vi "RePrint_Barcode.vi"(8 "error in":errorcluster, 9 "User Data":T1, 10 "RFID":string, 11 "Ref in":T2={"MS SQL Connection"=refnum, "UDL File"=path "", "Time"="", "DCODE"="", "WIP+1"=0, "MC No?"=0, "POKAYOKE?"=FALSE, "Expected Result"="", "Result [Status]"="", "Clock"=0.0, "RFID"="", "WIP Queue"=refnum, "TS Parameter"={"ProfitCenterCode"="", "LineCode"="", "WorkOrderNumber"="", "Model"="", "Model_with_Prefix"="", "VendorCode"="", "SetParameterDateCode"="", "PokaYoke"=0, "Target"=1, "Live_DateCode"="", "CustomerPartNumber"="", "Hand"="", "sBarcode"=FALSE, "FCA"=0, "Ent_Stamp"=timestamp(0 s since 1904-01-01), "STS_CD"=0.0}, "Data_Queue"=[], "RFID Serial No."=""} {"TS Parameter"."FCA" format="%01d"; "TS Parameter"."Target" min=1 max=100000; "TS Parameter"."PokaYoke" min=0 max=1}) -> (0 "error out":errorcluster, 2 "Barcode":string)   [LabVIEW 2020]
uses:
  Controls/TS_Parameter_V2.ctl
  Controls/TD SQL.ctl
  <vilib>/addons/database/Connection.llb/Conn ObjectReference.ctl
  Controls/WIP_State.ctl
  Controls/TS_Parameter.ctl
  Controls/user_log.ctl
  <vilib>/addons/database/Connection.llb/Conn Execute.vi
  MS SQL/MS_Global.vi
  <vilib>/addons/database/NI_Database_API.lvlib
panel:
  out "Total Seconds":i32
  out "TS Parameter":T5={"ProfitCenterCode"="", "LineCode"="", "WorkOrderNumber"="", "Model"="", "Model_with_Prefix"="", "VendorCode"="", "SetParameterDateCode"="", "PokaYoke"=0, "Target"=1, "Live_DateCode"="", "CustomerPartNumber"="", "Hose_Type"="", "sBarcode"=FALSE, "FCA"=0, "Ent_Stamp"=timestamp(0 s since 1904-01-01), "STS_CD"=0.0} {"FCA" format="%01d"; "Target" min=1 max=100000; "PokaYoke" min=0 max=1}
  out "text":string
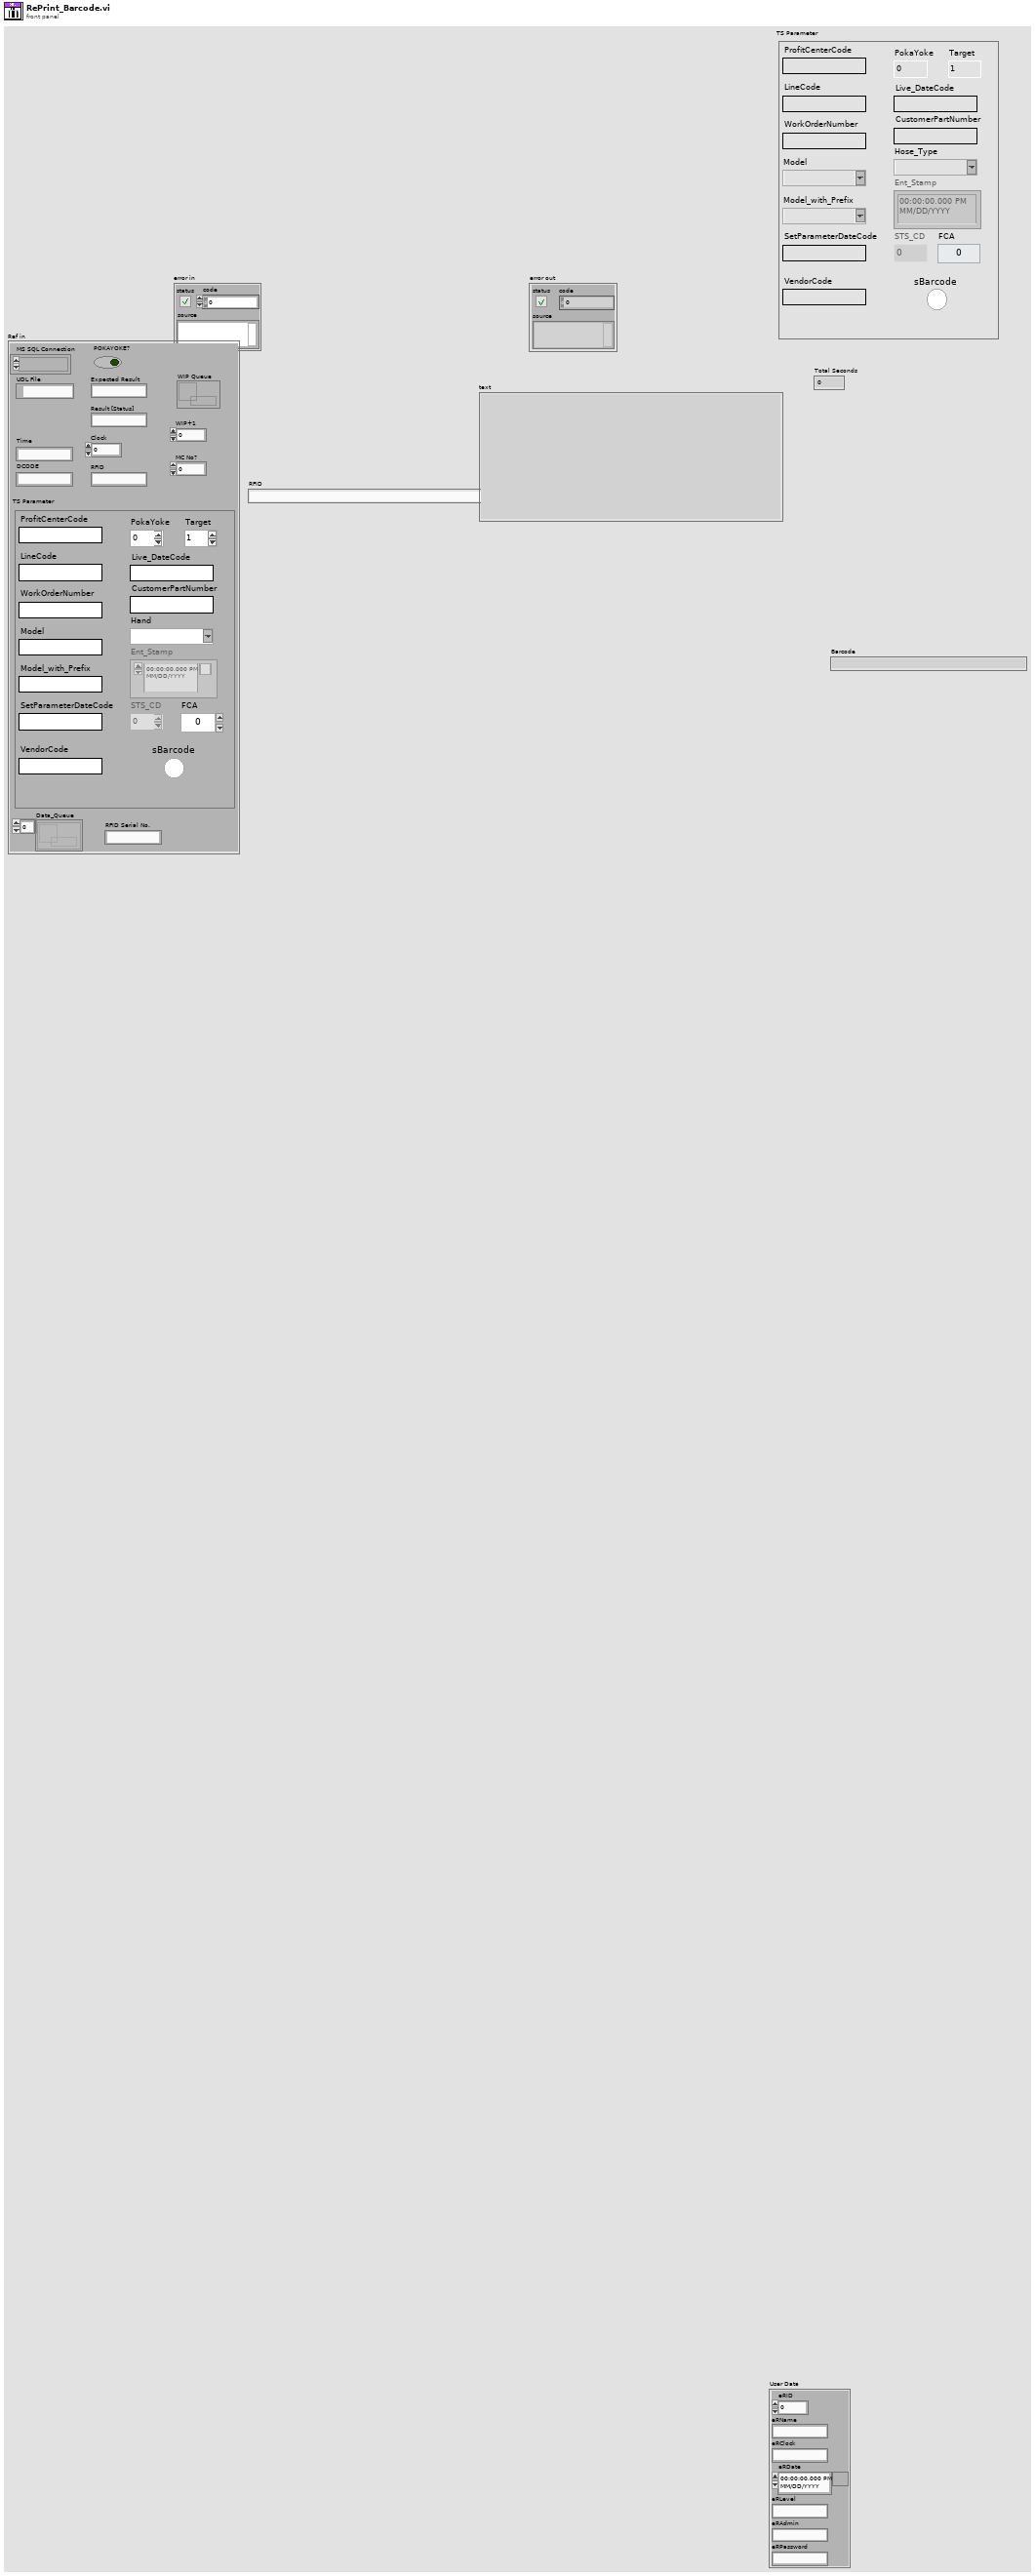
[diagram p1: front panel]
types:
  T1 = typedef "user_log.ctl" = cluster{"eRID":u16, "eRName":string, "eRClock":string, "eRDate":timestamp, "eRLevel":string, "eRAdmin":string, "eRPassword":string}
  T2 = typedef "TD SQL.ctl" = cluster{"MS SQL Connection":T3, "UDL File":path, "Time":string, "DCODE":string, "WIP+1":i64, "MC No?":i32, "POKAYOKE?":bool, "Expected Result":string, "Result [Status]":string, "Clock":dbl, "RFID":string, "WIP Queue":refnum<queue>, "TS Parameter":T4, "Data_Queue":refnum<queue>[], "RFID Serial No.":string}
  T3 = typedef "NI_Database_API.lvlib/Conn ObjectReference.ctl" = refnum<k1>
  T4 = typedef "TS_Parameter.ctl" = cluster{"ProfitCenterCode":string, "LineCode":string, "WorkOrderNumber":string, "Model":string, "Model_with_Prefix":string, "VendorCode":string, "SetParameterDateCode":string, "PokaYoke":i32, "Target":i32, "Live_DateCode":string, "CustomerPartNumber":string, "Hand":string, "sBarcode":bool, "FCA":i32, "Ent_Stamp":timestamp, "STS_CD":dbl}
  T5 = typedef "TS_Parameter_V2.ctl" = cluster{"ProfitCenterCode":string, "LineCode":string, "WorkOrderNumber":string, "Model":string, "Model_with_Prefix":string, "VendorCode":string, "SetParameterDateCode":string, "PokaYoke":i32, "Target":i32, "Live_DateCode":string, "CustomerPartNumber":string, "Hose_Type":string, "sBarcode":bool, "FCA":i32, "Ent_Stamp":timestamp, "STS_CD":dbl}
  T6 = enum16{"open", "replace", "create", "open or create", "replace or create", "replace or create with confirmation"}
  T7 = typedef "LVDateTimeRec.ctl" = cluster{"fractional second":dbl, "second":i32, "minute":i32, "hour":i32, "day of month":i32, "month":i32, "year":i32, "day of week":i32, "day of year":i32, "DST":i32}
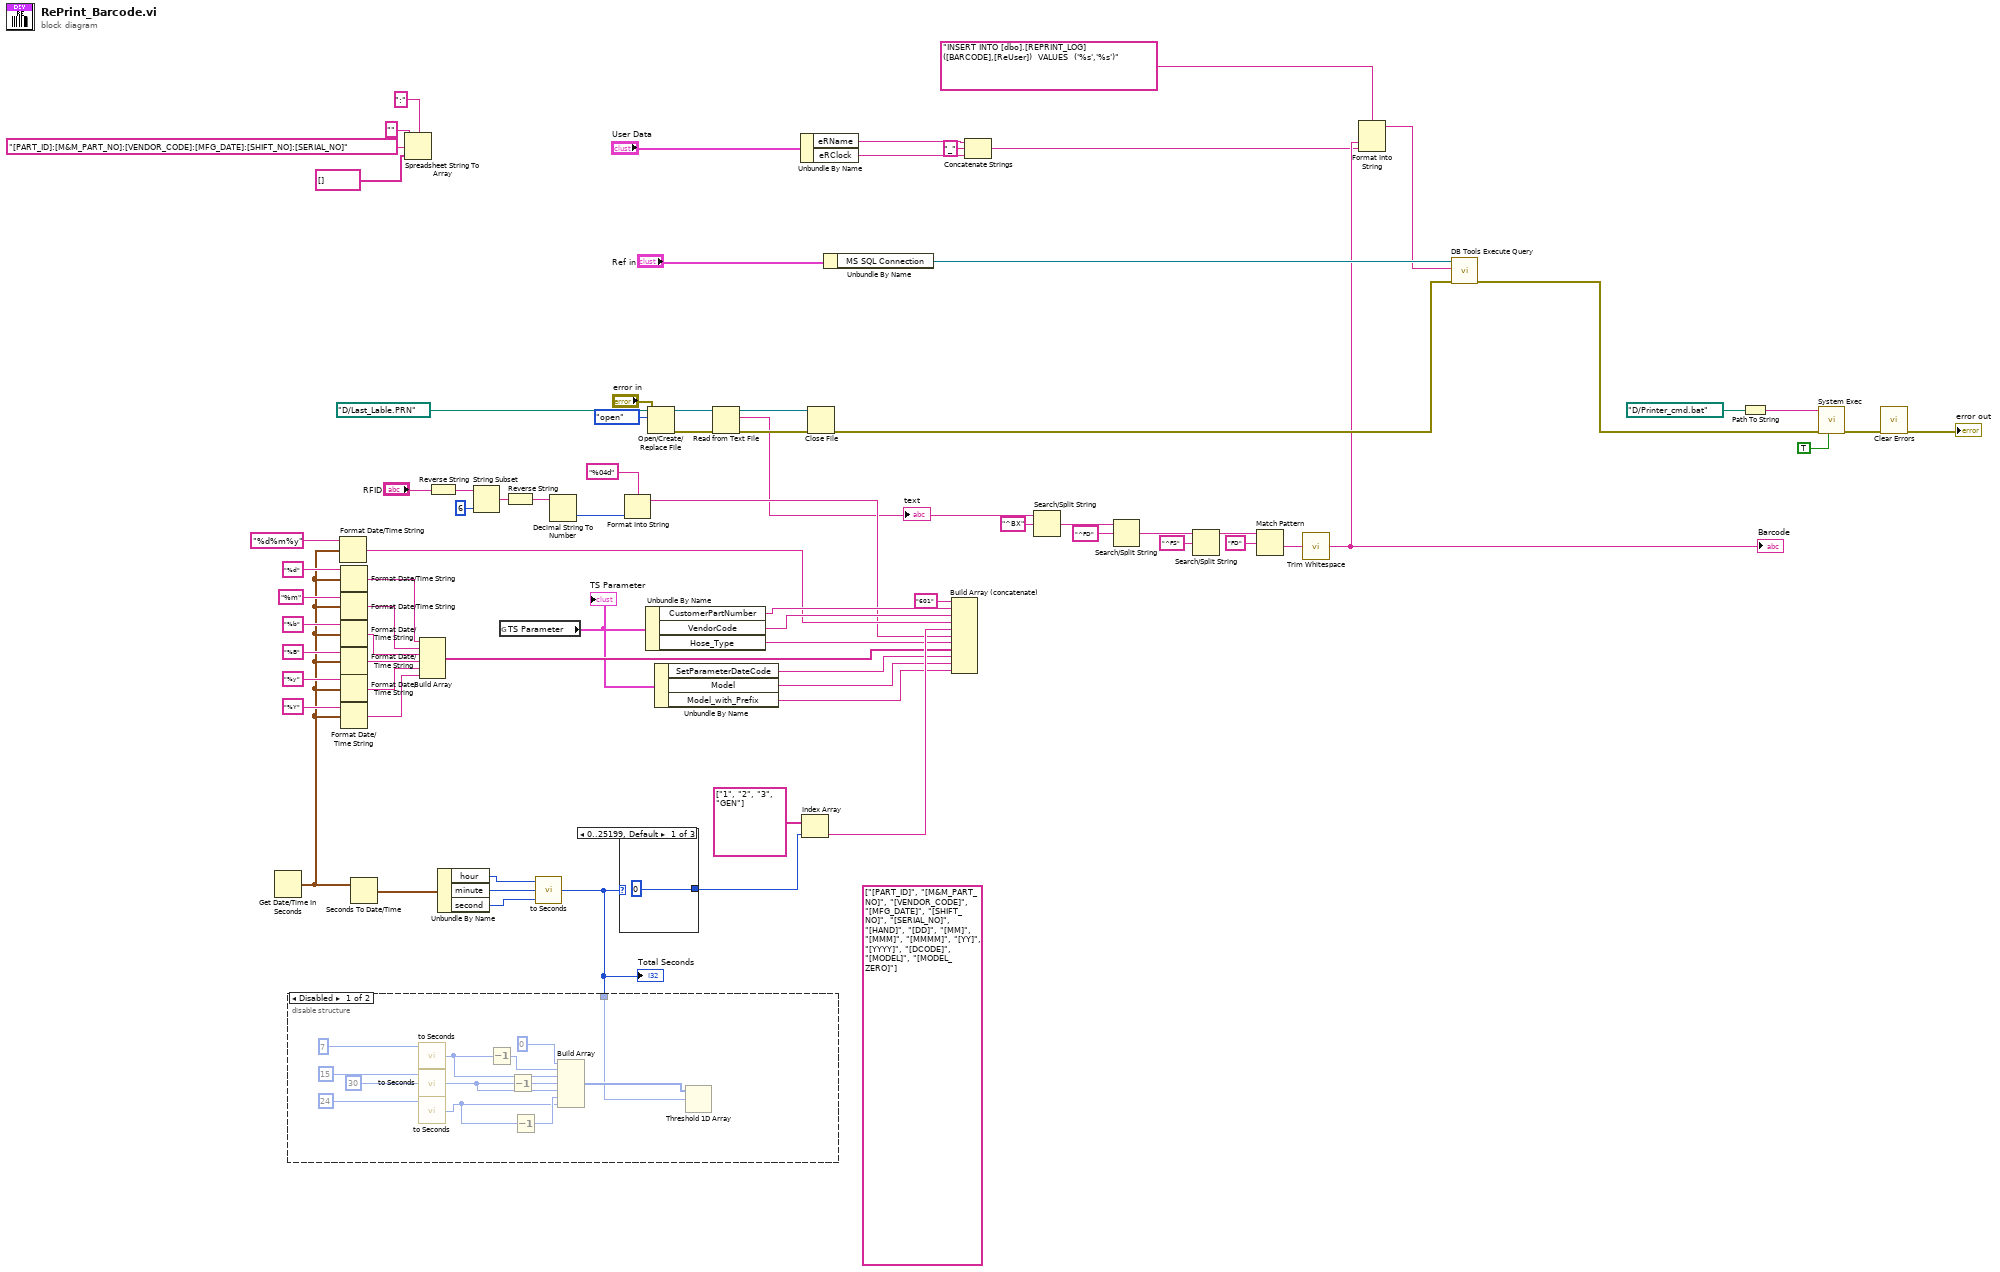
[diagram p0: block diagram]
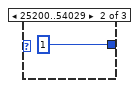
[diagram p3: hidden frame]
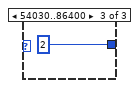
[diagram p4: hidden frame]
diagram:
  (unwired) string[] ["[PART_ID]", "[M&M_PART_NO]", "[VENDOR_CODE]", "[MFG_DATE]", "[SHIFT_NO]", "[SERIAL_NO]", "[HAND]", "[DD]", "[MM]", "[MMM]", "[MMMM]", "[YY]", "[YYYY]", "[DCODE]", "[MODEL]", "[MODEL_ZERO]"] ("array")
  n1 = Get Date/Time In Seconds() -> (seconds since 1Jan1904=w33:timestamp)
  n2 = Format Date/Time String(time format string (%c)="%d%m%y", seconds (now)=w33) -> (date/time string=w64:string)  [unwired: 1 in]
  n3 = Format Date/Time String(time format string (%c)="%d", seconds (now)=w33) -> (date/time string=w46:string)  [unwired: 1 in]
  n4 = Format Date/Time String(time format string (%c)="%m", seconds (now)=w33) -> (date/time string=w45:string)  [unwired: 1 in]
  n5 = Format Date/Time String(time format string (%c)="%b", seconds (now)=w33) -> (date/time string=w44:string)  [unwired: 1 in]
  n6 = Format Date/Time String(time format string (%c)="%B", seconds (now)=w33) -> (date/time string=w43:string)  [unwired: 1 in]
  n7 = Format Date/Time String(time format string (%c)="%y", seconds (now)=w33) -> (date/time string=w42:string)  [unwired: 1 in]
  n8 = Format Date/Time String(time format string (%c)="%Y", seconds (now)=w33) -> (date/time string=w41:string)  [unwired: 1 in]
  n9 = Seconds To Date/Time(time stamp (now)=w33) -> (date time rec=w39:T7)  [unwired: 1 in]
  n10 = Spreadsheet String To Array(delimiter (Tab)=":" ("spreadsheet string"), format string="", spreadsheet string="[PART_ID]:[M&M_PART_NO]:[VENDOR_CODE]:[MFG_DATE]:[SHIFT_NO]:[SERIAL_NO]", array type (2D Dbl)=string[] []) -> ()  [unwired: 1 out]
  n11 = Build Array(w46, w45, w44, w43, w42, w41) -> (w40:string[])
  n12 = Reverse String(1:"RFID") -> (0:w60:string)
  n13 = Unbundle By Name(w39) -> ("hour"=w38:i32, "minute"=w37:i32, "second"=w36:i32)
  n14 = String Subset(string=w60, length (rest)=6 ("length (rest)")) -> (substring=w58:string)  [unwired: 1 in]
  n15 = global read "MS_Global.vi" "TS Parameter"() -> (w4:T5)
  "TS Parameter" <- w4
  n16 = Reverse String(1:w58) -> (0:w57:string)
  n17 = call "to Seconds.vi"("Minute"=w36, "Second"=w37, "Hour"=w38) -> ("Total Seconds"=w35:i32)
  "Total Seconds" <- w35
  n18 = disable-structure shown="Disabled" {
    disable-tunnel: w35 -> [w78 _]
    frame Disabled {
      n19 = call "to Seconds.vi"("Hour"=7 ("length (rest)")) -> ("Total Seconds"=w84:i32)  [unwired: 2 in]
      n20 = call "to Seconds.vi"("Second"=30 ("length (rest)"), "Hour"=15 ("length (rest)")) -> ("Total Seconds"=w82:i32)  [unwired: 1 in]
      n21 = call "to Seconds.vi"("Hour"=24 ("length (rest)")) -> ("Total Seconds"=w79:i32)  [unwired: 2 in]
      n22 = Decrement(x=w84) -> (x-1=w83:i32)
      n23 = Decrement(x=w82) -> (x-1=w81:i32)
      n24 = Decrement(x=w79) -> (x-1=w80:i32)
      n25 = Build Array(0 ("element"), w83, w84, w81, w82, w80, w79) -> (w86:i32[])
      n26 = Threshold 1D Array(2:w78, 3:w86) -> ()  [unwired: 1 in, 1 out]
    }
    frame Enabled {
    }
  }
  n27 = Decimal String To Number(string=w57) -> (number=w56:i32)  [unwired: 2 in, 1 out]
  n28 = case shown="0..25199, Default" w35 {
    tunnel: [0 ("Total Seconds") 1 ("Total Seconds") 2 ("Total Seconds")] -> w34
    frame 0..25199, Default {
    }
    frame 25200..54029 {
    }
    frame 54030..86400 {
    }
  }
  n29 = Format Into String(format string="%04d", w56) -> (resulting string=w54:string)  [unwired: 2 in, 1 out]
  n30 = Unbundle By Name(w4) -> ("CustomerPartNumber"=w67:string, "VendorCode"=w66:string, "Hose_Type"=w53:string)
  n31 = Open/Create/Replace File(file path (use dialog)=path "D:/Last_Lable.PRN" ("appended path"), error in="error in", operation (0:open)=T6."open") -> (refnum out=w76:refnum<file>, error out=w77:errorcluster)  [unwired: 3 in, 1 out]
  n32 = Unbundle By Name(w4) -> ("SetParameterDateCode"=w3:string, "Model"=w2:string, "Model_with_Prefix"=w1:string)
  n33 = Read from Text File(file (use dialog)=w76, error in=w77) -> (refnum out=w75:refnum<file>, text=w20:string, error out=w74:errorcluster)  [unwired: 2 in, 1 out]
  "text" <- w20
  n34 = Unbundle By Name("User Data") -> ("eRName"=w11:string, "eRClock"=w10:string)
  n35 = Index Array(array=string[] ["1", "2", "3", "GEN"], index=w34) -> (element=w62:string)
  n36 = Close File(refnum=w75, error in=w74) -> (error out=w15:errorcluster)  [unwired: 1 out]
  n37 = Unbundle By Name("Ref in") -> ("MS SQL Connection"=w16:T3)
  n38 = Build Array (concatenate)("601" ("spreadsheet string"), w67, w66, w64, w62, w54, w53, w40, w3, w2, w1) -> ()  [unwired: 1 out]
  n39 = Concatenate Strings(w11, "_" ("string"), w10) -> (w6:string)
  n40 = Search/Split String(string=w20, search string/char (-)="^BX" ("regular expression")) -> (match + rest of string=w29:string)  [unwired: 1 in, 2 out]
  n41 = Search/Split String(string=w29, search string/char (-)="^FD" ("regular expression")) -> (match + rest of string=w28:string)  [unwired: 1 in, 2 out]
  n42 = Search/Split String(string=w28, search string/char (-)="^FS" ("regular expression")) -> (substring before match=w25:string)  [unwired: 1 in, 2 out]
  n43 = Match Pattern(string=w25, regular expression="FD") -> (after substring=w23:string)  [unwired: 1 in, 3 out]
  n44 = call <vilib>:"Trim Whitespace.vi"("string"=w23) -> ("trimmed string"=w7:string)  [unwired: 1 in]
  "Barcode" <- w7
  n45 = Format Into String(format string="INSERT INTO [dbo].[REPRINT_LOG] ([BARCODE],[ReUser])  VALUES  ('%s','%s')" ("SQL query"), w7, w6) -> (resulting string=w5:string)  [unwired: 2 in, 1 out]
  n46 = call-poly <vilib>:"DB Tools Execute Query.vi"("error in (no error)"=w15, "SQL query"=w5, "connection reference"=w16) -> ("error out"=w14:errorcluster)  [unwired: 5 in, 1 out]
  n47 = Path To String(path=path "D:/Printer_cmd.bat" ("appended path")) -> (string=w30:string)
  n48 = call <vilib>:"System Exec.vi"("run minimized? (F)"=TRUE, "error in (no error)"=w14, "command line"=w30) -> ("error out"=w19:errorcluster)  [unwired: 5 in, 3 out]
  n49 = call <vilib>:"Clear Errors.vi"("error in (no error)"=w19) -> ("error out"=→"error out":errorcluster)  [unwired: 5 in, 1 out]
